vi "Format Indented.vi"(9 "Depth":i32, 10 "New Line needed":bool, 11 "Text":string) -> (3 "Indented Text":string)   [LabVIEW 2020, in "JSONtext.lvlib"]
uses:
  <vilib>/JDP Science/JSONtext/JSONtext.lvlib
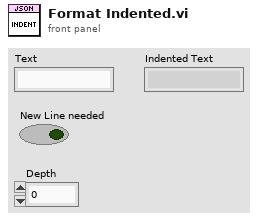
[diagram p1: front panel]
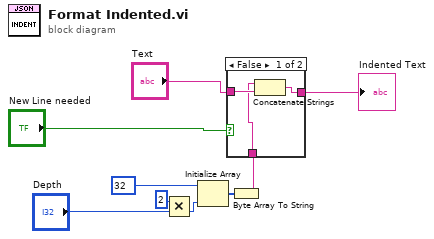
[diagram p0: block diagram]
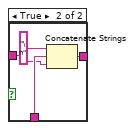
[diagram p2: hidden frame]
diagram:
  n1 = Multiply(x=2, y="Depth") -> (x*y=w7:i32)
  n2 = Initialize Array(u8 32, w7) -> (w4:u8[])
  n3 = Byte Array To String(unsigned byte array=w4) -> (string=w5:string)
  n4 = case shown="False" "New Line needed" {
    tunnel: "Text" -> [w12 w13]
    tunnel: [w11 w16] -> w1
    tunnel: w5 -> [w10 w14]
    frame False {
      n5 = Concatenate Strings(w10, w12) -> (w11:string)
    }
    frame True {
      n6 = Concatenate Strings("\n" ("string"), w14, w13) -> (w16:string)
    }
  }
  "Indented Text" <- w1
